vi "GetRandomData.vi"(0 "显示界面":T1) -> ()   [LabVIEW 2019]
uses:
  ctl/Display.ctl
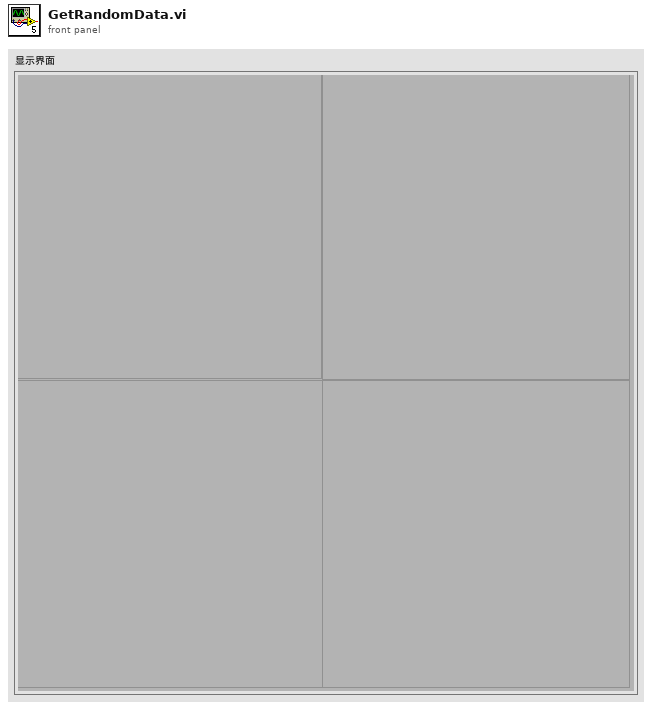
[diagram p1: front panel]
types:
  T1 = typedef "Display.ctl" = cluster{"左上":bool, "右上":bool, "左下":bool, "右下":bool}
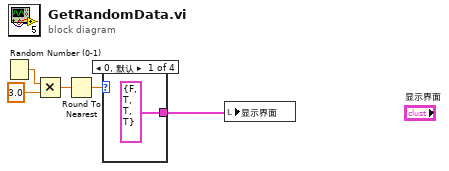
[diagram p0: block diagram]
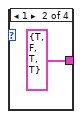
[diagram p2: hidden frame]
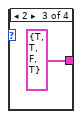
[diagram p3: hidden frame]
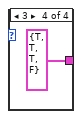
[diagram p4: hidden frame]
diagram:
  n1 = Random Number (0-1)() -> (number: 0 to 1=w5:dbl)
  n2 = Multiply(x=w5, y=3.0) -> (x*y=w3:dbl)
  n3 = Round To Nearest(number=w3) -> (nearest integer value=w2:dbl)
  n4 = case shown="0, 默认" w2 {
    tunnel: [T1 {"左上"=FALSE, "右上"=TRUE, "左下"=TRUE, "右下"=TRUE} ("显示界面") T1 {"左上"=TRUE, "右上"=FALSE, "左下"=TRUE, "右下"=TRUE} ("显示界面") T1 {"左上"=TRUE, "右上"=TRUE, "左下"=FALSE, "右下"=TRUE} ("显示界面") T1 {"左上"=TRUE, "右上"=TRUE, "左下"=TRUE, "右下"=FALSE} ("显示界面")] -> w1
    frame 0, Default {
    }
    frame 1 {
    }
    frame 2 {
    }
    frame 3 {
    }
  }
  n5 = local write "显示界面"(w1) -> ()
